vi "SettingsFiles.vi"(8 "pattern":string, 11 "settings file name":string) -> (0 "filenames":string[](array[string]), 3 "file path":path)   [LabVIEW 2022 SP3]
uses:
  <vilib>/Utility/error.llb/Trim Whitespace One-Sided.vi
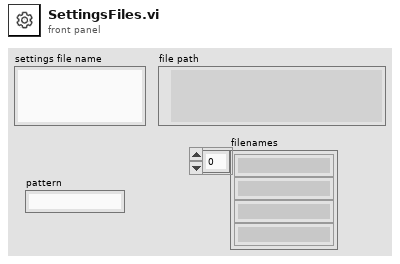
[diagram p1: front panel]
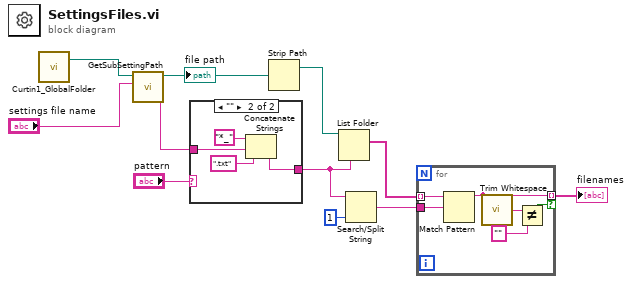
[diagram p0: block diagram]
diagram:
  n1 = call "Curtin1_GlobalFolder.vi"() -> ("LabVIEW Data Path"=w5:path)  [unwired: 1 in, 1 out]
  n2 = call "GetSubSettingPath.vi"("settings file name"="settings file name", "LabVIEW Data Path"=w5) -> ("folder"=w1:string, "settings file path"=w3:path)  [unwired: 8 in]
  "file path" <- w3
  n3 = case shown="\"\"" "pattern" {
    selector: "pattern" -> [w12 _]
    tunnel: w1 -> [_ w15]
    tunnel: [w12 w14] -> w9
    frame Default {
    }
    frame "" {
      n4 = Concatenate Strings("*_" ("pattern"), w15, ".txt" ("pattern")) -> (w14:string)
    }
  }
  n5 = Strip Path(path=w3) -> (stripped path=w2:path)  [unwired: 1 out]
  n6 = List Folder(path=w2, pattern=w9) -> (filenames=w10:string[])  [unwired: 2 in, 3 out]
  n7 = Search/Split String(string=w9, offset (0)=1) -> (match + rest of string=w7:string)  [unwired: 1 in, 2 out]
  n8 = for {
    tunnel: w10 -> [w22] mode=indexing
    tunnel: w7 -> [w21]
    tunnel: [w20] -> w6 mode=indexing if=w17
    n9 = Match Pattern(string=w22, regular expression=w21) -> (before substring=w20:string)  [unwired: 1 in, 3 out]
    n10 = call <vilib>:"Trim Whitespace.vi"("string"=w20) -> ("trimmed string"=w19:string)  [unwired: 1 in]
    n11 = Not Equal?(x=w19, y="") -> (x != y?=w17:bool)
  }
  "filenames" <- w6
